vi "TEMP.vi"() -> ()   [LabVIEW 2017]
uses:
  <vilib>/addons/InsightCM/MessageBus/Base/controls/DataEvent.ctl
  <vilib>/addons/InsightCM/MessageBus/Base/controls/KeyValuePair.ctl
  <vilib>/addons/InsightCM/MessageBus/MessageService/IcmMessageService.lvclass
panel:
  out "Output":T1(array[cluster])
  in  "Input: trend id 2":string="5cf73d1ba0991c03a125caf0"
  in  "Input: sensor ID":string="5cf73d1ba0991c03a125caee"
  out "Array":T2(array[cluster])=[{"Id"="{6C8D9120-E97A-11E9-9C35-00802F195E7B}", "Timestamp"=1570418361, "Value"=0.0018771609136779158}, {"Id"="{7F637499-E981-11E9-A30F-00802F195E7B}", "Timestamp"=1570421399, "Value"=0.0018826798587614586}, {"Id"="{E4F320D8-E982-11E9-A025-00802F195E7B}", "Timestamp"=1570421999, "Value"=0.0018771413916787638}, {"Id"="{97B5DB2B-E983-11E9-8698-00802F195E7B}", "Timestamp"=1570422299, "Value"=0.0018758608022062296}, {"Id"="{FD7A4AB0-E984-11E9-A552-00802F195E7B}", "Timestamp"=1570422899, "Value"=0.0018778648123666678}, {"Id"="{B025F119-E985-11E9-9683-00802F195E7B}", "Timestamp"=1570423199, "Value"=0.0018708454227732057}, {"Id"="{62F87800-E986-11E9-9683-00802F195E7B}", "Timestamp"=1570423499, "Value"=0.0018792979598656902}]
  in  "Input: trend id":string="5cf73d1ba0991c03a125caef"
  out "DataEvents":T3[](array[typedef])=[{"Id"="{6C8D9120-E97A-11E9-9C35-00802F195E7B}", "AssetNodeId"="5cf73cf3a0991c03a125caeb", "Timestamp"=1570418361, "Props"=[{"Key"="DeviceName", "Value"="John-9068"}, {"Key"="DataGroup", "Value"="Equipment"}, {"Key"="OpState", "Value"="Default"}, {"Key"="Reason", "Value"="User Event"}, {"Key"="HighRate", "Value"="true"}, {"Key"="HasDataSets", "Value"="true"}]}, {"Id"="{7F637499-E981-11E9-A30F-00802F195E7B}", "AssetNodeId"="5cf73cf3a0991c03a125caeb", "Timestamp"=1570421399, "Props"=[{"Key"="DeviceName", "Value"="John-9068"}, {"Key"="DataGroup", "Value"="Equipment"}, {"Key"="OpState", "Value"="Default"}, {"Key"="Reason", "Value"="Periodic Event"}, {"Key"="HighRate", "Value"="true"}, {"Key"="HasDataSets", "Value"="true"}]}, {"Id"="{E4F320D8-E982-11E9-A025-00802F195E7B}", "AssetNodeId"="5cf73cf3a0991c03a125caeb", "Timestamp"=1570421999, "Props"=[{"Key"="DeviceName", "Value"="John-9068"}, {"Key"="DataGroup", "Value"="Equipment"}, {"Key"="OpState", "Value"="Default"}, {"Key"="Reason", "Value"="Periodic Event"}, {"Key"="HighRate", "Value"="true"}, {"Key"="HasDataSets", "Value"="true"}]}, {"Id"="{97B5DB2B-E983-11E9-8698-00802F195E7B}", "AssetNodeId"="5cf73cf3a0991c03a125caeb", "Timestamp"=1570422299, "Props"=[{"Key"="DeviceName", "Value"="John-9068"}, {"Key"="DataGroup", "Value"="Equipment"}, {"Key"="OpState", "Value"="Default"}, {"Key"="Reason", "Value"="Periodic Event"}, {"Key"="HighRate", "Value"="true"}, {"Key"="HasDataSets", "Value"="true"}]}, {"Id"="{FD7A4AB0-E984-11E9-A552-00802F195E7B}", "AssetNodeId"="5cf73cf3a0991c03a125caeb", "Timestamp"=1570422899, "Props"=[{"Key"="DeviceName", "Value"="John-9068"}, {"Key"="DataGroup", "Value"="Equipment"}, {"Key"="OpState", "Value"="Default"}, {"Key"="Reason", "Value"="Periodic Event"}, {"Key"="HighRate", "Value"="true"}, {"Key"="HasDataSets", "Value"="true"}]}, {"Id"="{B025F119-E985-11E9-9683-00802F195E7B}", "AssetNodeId"="5cf73cf3a0991c03a125caeb", "Timestamp"=1570423199, "Props"=[{"Key"="DeviceName", "Value"="John-9068"}, {"Key"="DataGroup", "Value"="Equipment"}, {"Key"="OpState", "Value"="Default"}, {"Key"="Reason", "Value"="Periodic Event"}, {"Key"="HighRate", "Value"="true"}, {"Key"="HasDataSets", "Value"="true"}]}, {"Id"="{62F87800-E986-11E9-9683-00802F195E7B}", "AssetNodeId"="5cf73cf3a0991c03a125caeb", "Timestamp"=1570423499, "Props"=[{"Key"="DeviceName", "Value"="John-9068"}, {"Key"="DataGroup", "Value"="Equipment"}, {"Key"="OpState", "Value"="Default"}, {"Key"="Reason", "Value"="Periodic Event"}, {"Key"="HighRate", "Value"="true"}, {"Key"="HasDataSets", "Value"="true"}]}]
  in  "End Time":timestamp=timestamp(3653268533.6102896 s since 1904-01-01)
  in  "Start Time":timestamp=timestamp(3653222452.61 s since 1904-01-01)
  in  "Input: Asset id":string="5cf73cf3a0991c03a125caeb"
  # "Equipment"
  # "First sensor"
  # "5cf73d1ba0991c03a125caee"
  # "Crest factor"
  # "Derived Peak"
  # "5cf73d1ba0991c03a125caee"
  # "5cf73d32a0991c03a125cafc"
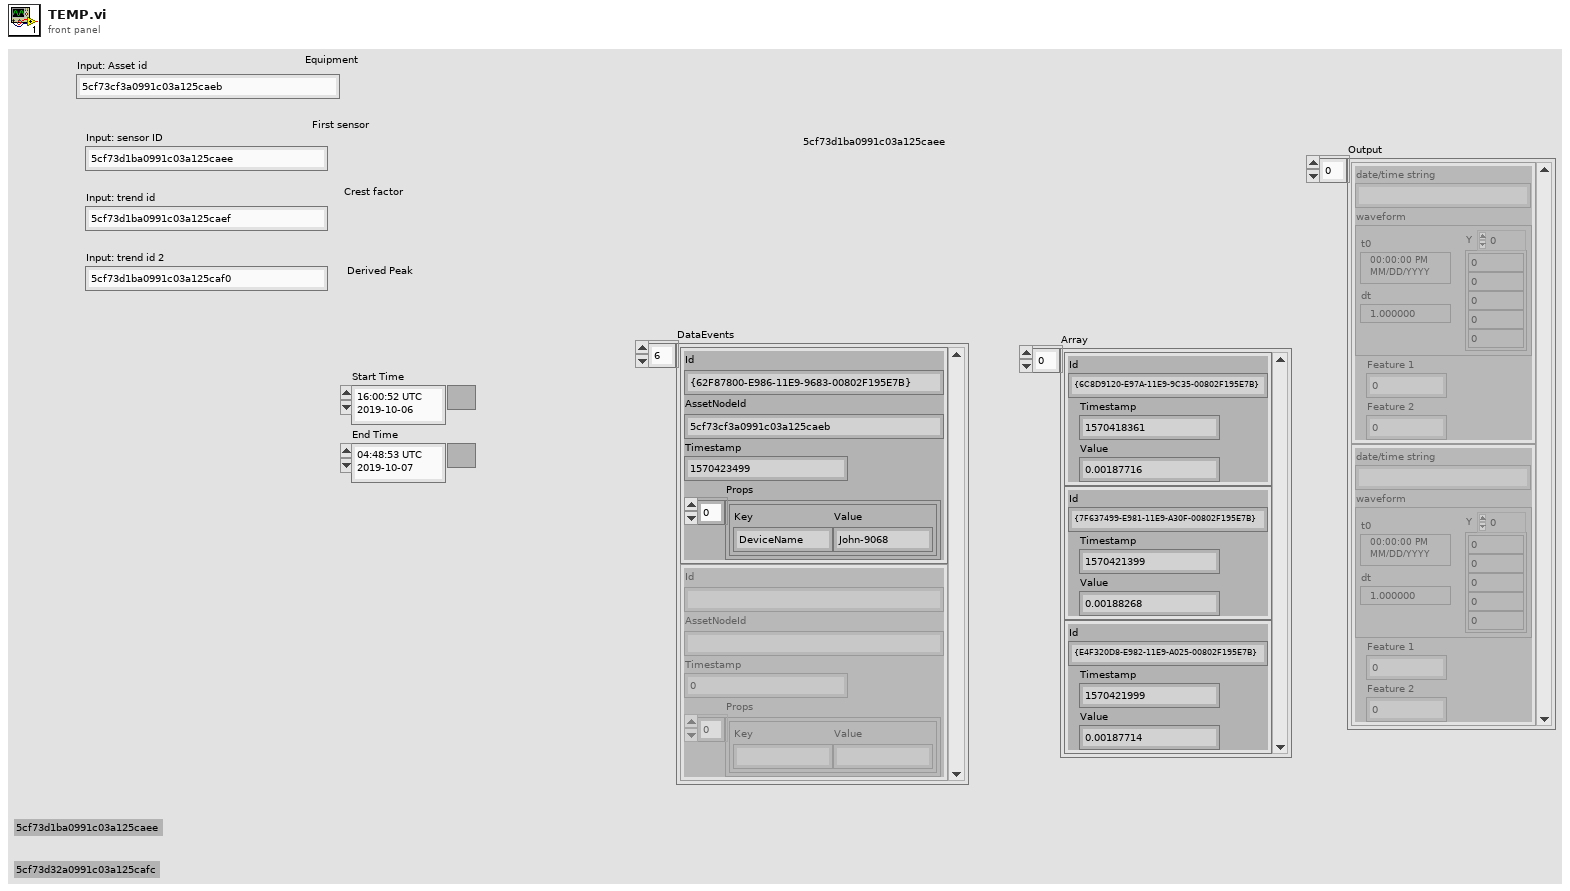
[diagram p1: front panel]
types:
  T1 = cluster{"date/time string":string, "waveform":waveform(sgl), "Feature 1":dbl, "Feature 2":dbl}[]
  T2 = cluster{"Id":string, "Timestamp":i64, "Value":dbl}[]
  T3 = typedef "DataEvent.ctl" = cluster{"Id":string, "AssetNodeId":string, "Timestamp":i64, "Props":T4[]}
  T4 = typedef "KeyValuePair.ctl" = cluster{"Key":string, "Value":string}
  T5 = typedef "TrendPoint.ctl" = cluster{"TrendPointId":string, "DataEventId":string, "Timestamp":i64, "Value":dbl, "Props":T4[]}
  T6 = typedef "DataSetByteData.ctl" = cluster{"Id":string, "DataEventId":string, "AssetNodeId":string, "Type":string, "T0":i64, "Props":T4[], "DataBase64":string}
  T7 = cluster{"date/time string":string, "waveform":waveform(sgl), "Value":dbl, "Value":dbl}
  T8 = cluster{"Id":void, "Timestamp":void, "Value":dbl}
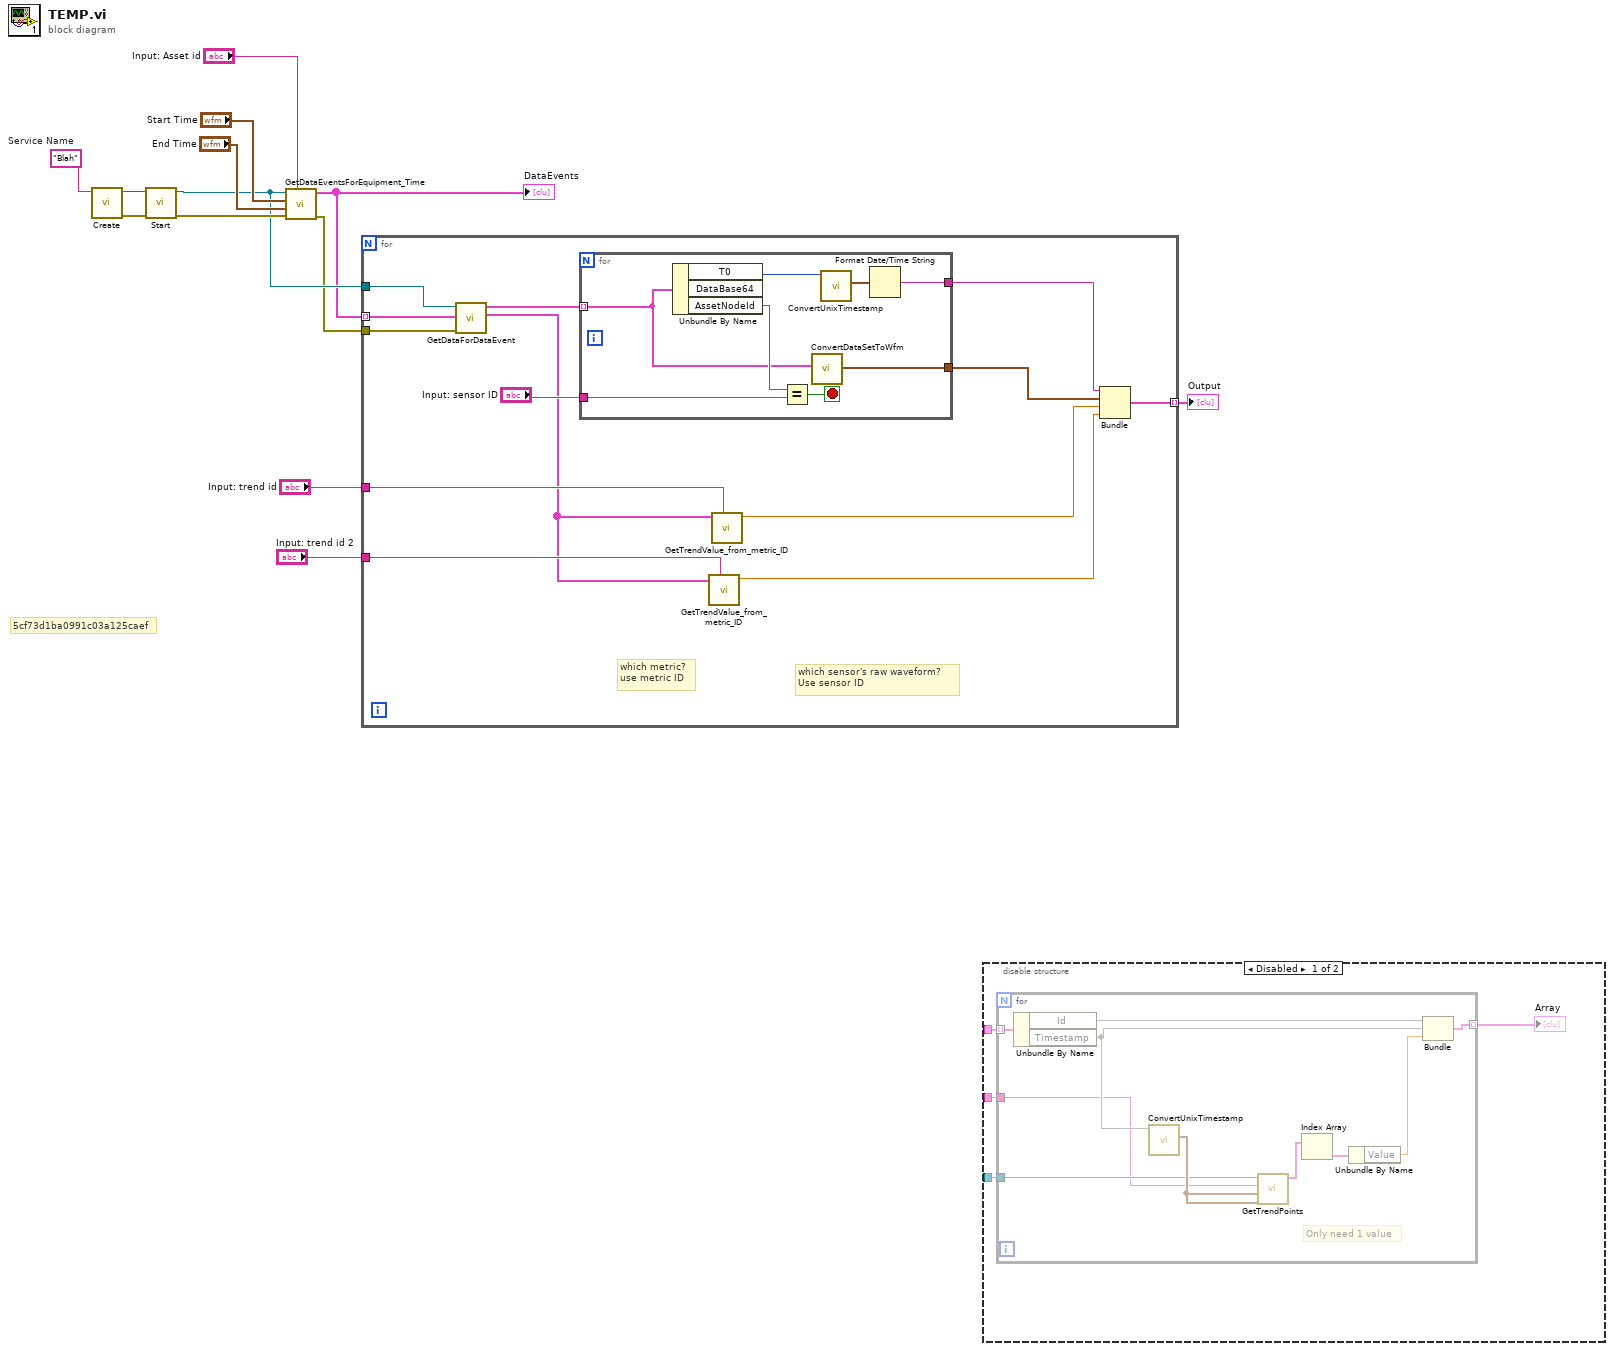
[diagram p0: block diagram]
diagram:
  w13 = "Blah"  # Service Name
  # "5cf73d1ba0991c03a125caef"
  n1 = call <vilib>:"Create.vi"("service name"=w13) -> ("error out"=w11:errorcluster, "service out"=w12:refnum<class "IcmMessageService.lvclass">)  [unwired: 9 in]
  n2 = call <vilib>:"Start.vi"("error in (no error)"=w11, "service in"=w12) -> ("error out"=w10:errorcluster, "service out"=w6:refnum<class "IcmMessageService.lvclass">)  [unwired: 8 in]
  n3 = call "GetDataEventsForEquipment_Time.vi"("equipment id"="Input: Asset id", "error in (no error)"=w10, "End Time"="End Time", "Start Time"="Start Time", "service"=w6) -> ("error out"=w5:errorcluster, "DataEvents"=w4:T3[])  [unwired: 5 in]
  "DataEvents" <- w4
  n4 = for {
    tunnel: w6 -> [w26]
    tunnel: w5 -> [w25]
    tunnel: w4 -> [w24] mode=indexing
    tunnel: [w19] -> w1 mode=indexing
    tunnel: "Input: trend id" -> [w17]
    tunnel: "Input: trend id 2" -> [w16]
    # "which metric?\nuse metric ID"
    # "which sensor's raw waveform?\nUse sensor ID"
    n5 = call "GetDataForDataEvent.vi"("error in (no error)"=w25, "DataEvent"=w24, "service"=w26) -> ("TrendPoints"=w15:T5[], "DataSets"=w23:T6[])  [unwired: 6 in, 1 out]
    n6 = for {
      tunnel: w23 -> [w29] mode=indexing
      tunnel: "Input: sensor ID" -> [w33]
      tunnel: [w28] -> w22
      tunnel: [w27] -> w21
      stop <- w32 stop-if-true
      n7 = Unbundle By Name(w29) -> ("T0"=w30:i64, "AssetNodeId"=w34:string)  [unwired: 1 out]
      n8 = Equal?(x=w34, y=w33) -> (x = y?=w32:bool)
      n9 = call "ConvertDataSetToWfm.vi"("DataSet"=w29) -> ("waveform"=w27:waveform(sgl))  [unwired: 10 in]
      n10 = call <vilib>:"ConvertUnixTimestamp.vi"("Timestamp in"=w30) -> ("Time Stamp out"=w31:timestamp)  [unwired: 10 in]
      n11 = Format Date/Time String(seconds (now)=w31) -> (date/time string=w28:string)  [unwired: 2 in]
    }
    n12 = call "GetTrendValue_from_metric_ID.vi"("Input: trend id"=w16, "TrendPoints"=w15) -> ("Value"=w14:dbl)  [unwired: 9 in]
    n13 = call "GetTrendValue_from_metric_ID.vi"("Input: trend id"=w17, "TrendPoints"=w15) -> ("Value"=w20:dbl)  [unwired: 9 in]
    n14 = Bundle("date/time string"=w22, "waveform"=w21, "Value"=w20, "Value"=w14) -> (w19:T7)  [unwired: 1 in]
  }
  "Output" <- w1
  n15 = disable-structure shown="Disabled" {
    disable-tunnel: _ -> [w38 _]
    disable-tunnel: _ -> [w37 _]
    disable-tunnel: _ -> [w36 _]
    frame Disabled {
      n16 = for {
        tunnel: w38 -> [w48] mode=indexing
        tunnel: [w46] -> w35 mode=indexing
        tunnel: w37 -> [w43]
        tunnel: w36 -> [w42]
        # "Only need 1 value"
        n17 = Unbundle By Name(w48) -> ("Id"=w47, "Timestamp"=w45)
        n18 = call <vilib>:"ConvertUnixTimestamp.vi"("Timestamp in"=w45) -> ("Time Stamp out"=w44:timestamp)  [unwired: 10 in]
        n19 = call "GetTrendPoints.vi"("End Time"=w44, "Start Time"=w44, "trend id"=w42, "service"=w43) -> ("TrendPoints"=w41:T5[])  [unwired: 6 in, 1 out]
        n20 = Index Array(array=w41) -> (element=w40:T5)  [unwired: 1 in]
        n21 = Unbundle By Name(w40) -> ("Value"=w39:dbl)
        n22 = Bundle("Id"=w47, "Timestamp"=w45, "Value"=w39) -> (w46:T8)  [unwired: 1 in]
      }
      "Array" <- w35
    }
    frame Enabled {
    }
  }
